vi "Accumulated heat Loss.vi"(10 "Coord":cluster{"Row":i32, "Col":i32}, 11 "Proto in":refnum<class "Heat Map.lvclass">) -> (2 "Min Heat":i32, 3 "Proto out":refnum<class "Heat Map.lvclass">)   [LabVIEW 2021, in "Heat Map.lvclass"]
uses:
  Heat Map.lvclass
  Heat Map.lvclass/Heat Map.ctl
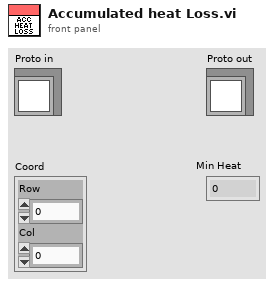
[diagram p1: front panel]
types:
  T1 = typedef "Heat Map.lvclass/Direction.ctl" = enum16{"Up", "Down", "Right", "Left"}
  T2 = map{cluster{"Row":i32, "Col":i32}, set{cluster{"Heat":i32, "Prev Steps":T1[]}}}
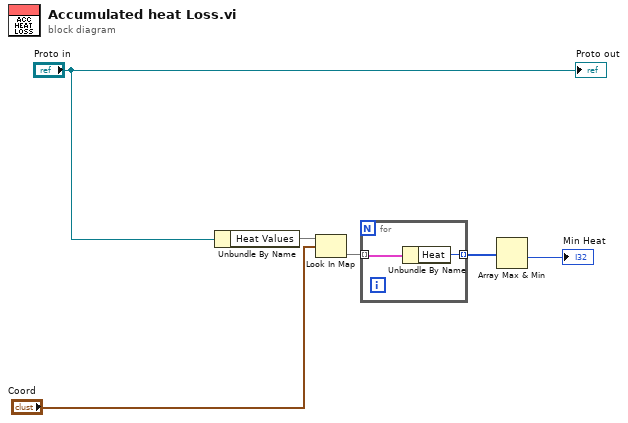
[diagram p0: block diagram]
diagram:
  n1 = Unbundle By Name("Proto in") -> ("Heat Values"=w6:T2)
  n2 = Look In Map(map=w6, key="Coord") -> (value=w4:set{cluster{"Heat":i32, "Prev Steps":T1[]}})  [unwired: 1 in, 1 out]
  n3 = for {
    tunnel: w4 -> [w8] mode=indexing
    tunnel: [w7] -> w3 mode=indexing
    n4 = Unbundle By Name(w8) -> ("Heat"=w7:i32)
  }
  n5 = Array Max & Min(array=w3) -> (min value=→"Min Heat":i32)  [unwired: 3 out]
  "Proto out" <- "Proto in"
